vi "HexStringToU32.vi"(0 "Input String":string, 7 "Starting Offset":i32) -> (4 "Number Out":u32)   [LabVIEW 2014]
doc: "Takes an input from \"String Input\" in the form of a 32-bit integer with spaces between bytes starting at \"Starting Offset\" and converts it to a U32 integer output, \"Number Out.\""
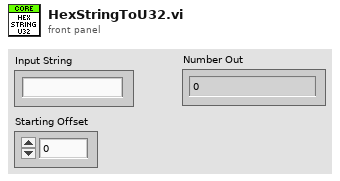
[diagram p1: front panel]
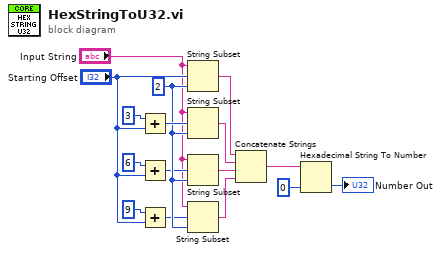
[diagram p0: block diagram]
diagram:
  w9 = 2 ("offset (0)")
  n1 = Add(x=3, y="Starting Offset") -> (x+y=w10:i32)
  n2 = Add(x=6, y="Starting Offset") -> (x+y=w6:i32)
  n3 = Add(x=9, y="Starting Offset") -> (x+y=w5:i32)
  n4 = String Subset(string="Input String", offset (0)="Starting Offset", length (rest)=w9) -> (substring=w14:string)
  n5 = String Subset(string="Input String", offset (0)=w10, length (rest)=w9) -> (substring=w13:string)
  n6 = String Subset(string="Input String", offset (0)=w6, length (rest)=w9) -> (substring=w2:string)
  n7 = String Subset(string="Input String", offset (0)=w5, length (rest)=w9) -> (substring=w1:string)
  n8 = Concatenate Strings(w14, w13, w2, w1) -> (w16:string)
  n9 = Hexadecimal String To Number(string=w16, default (0uL)=u32 0) -> (number=→"Number Out":u32)  [unwired: 1 in, 1 out]
